vi "Coordinator (SubVI).vi"(6 "mV per step":dbl, 7 "Numeric 3":dbl, 9 "Numeric 5":dbl, 10 "Numeric 4":dbl, 11 "Numeric 6":dbl) -> (2 "Numeric 2":dbl, 3 "Numeric":dbl)   [LabVIEW 2024]
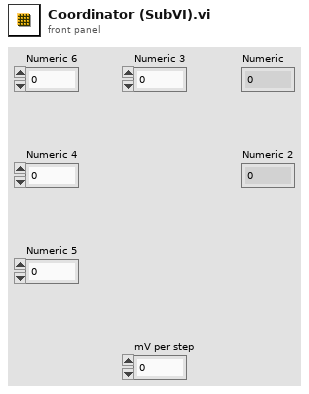
[diagram p1: front panel]
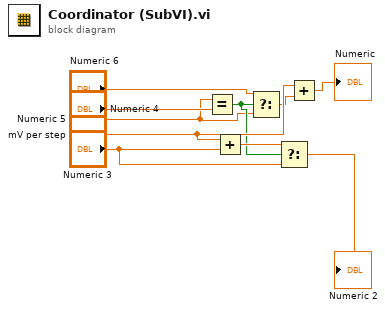
[diagram p0: block diagram]
diagram:
  n1 = Equal?(x="Numeric 5", y="Numeric 4") -> (x = y?=w5:bool)
  n2 = Add(x="mV per step", y="Numeric 3") -> (x+y=w6:dbl)
  n3 = Select(t="Numeric 6", s=w5, f="Numeric 5") -> (s? t:f=w4:dbl)
  n4 = Select(t=w6, s=w5, f="Numeric 3") -> (s? t:f=→"Numeric 2":dbl)
  n5 = Add(x="mV per step", y=w4) -> (x+y=→"Numeric":dbl)
